vi "Get Software Version.vi"(0 "eprom":u32, 1 "dllrev":u32, 5 "coffile":u32, 7 "vxdrev":u32, 9 "vxdver":u32, 12 "dllver":u32) -> (2 "function return":u32, 3 "dllrev out":u32, 4 "eprom out":u32, 6 "coffile out":u32, 8 "vxdrev out":u32, 10 "vxdver out":u32, 14 "dllver out":u32)   [LabVIEW 2018, in "AndorSDK.lvlib"]
doc: "EXPNETTYPE unsigned int WINAPI GetSoftwareVersion(unsigned int * eprom, unsigned int * coffile, unsigned int * vxdrev, unsigned int * vxdver, unsigned int * dllrev, unsigned int * dllver);"
uses:
  AndorSDK.lvlib
  ATMCD32D.dll
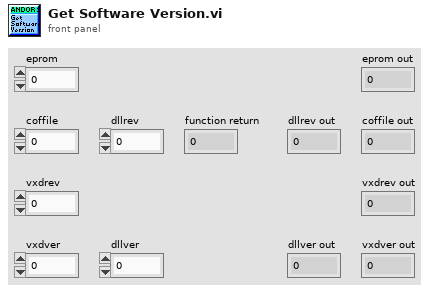
[diagram p1: front panel]
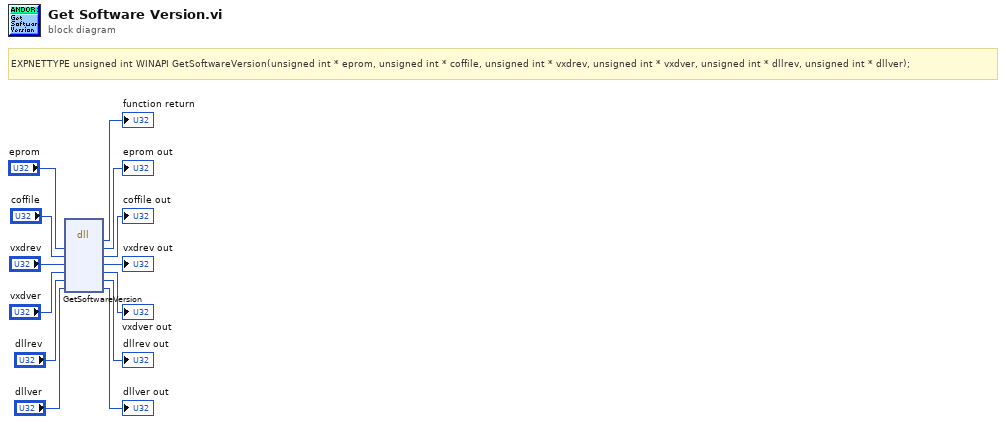
[diagram p0: block diagram]
diagram:
  # "EXPNETTYPE unsigned int WINAPI GetSoftwareVersion(unsigned int * eprom, unsigned int * coffile, unsigned int * vxdrev, unsigned int * vxdver, unsigned int * dllrev, unsigned int * dllver);"
  n1 = dll-call lib="PTH2babs E\nPersönliches02 - Arbeit03-HiwijobsLabviewCodelibANDOR\tAndor SDK\nATMCD32D.*" fn="GetSoftwareVersion"("eprom"="eprom", "coffile"="coffile", "vxdrev"="vxdrev", "vxdver"="vxdver", "dllrev"="dllrev", "dllver"="dllver") -> (→"function return":u32, "eprom"=→"eprom out":u32, "coffile"=→"coffile out":u32, "vxdrev"=→"vxdrev out":u32, "vxdver"=→"vxdver out":u32, "dllrev"=→"dllrev out":u32, "dllver"=→"dllver out":u32)  [unwired: 3 in, 2 out]
